vi "sprite.vi"() -> ()   [LabVIEW 2023]
uses:
  data_type/pixel/pixel.ctl
panel:
  in  "mutiply by":u64 min=1 step=1
  in  "exclude color":u32(colorbox)
  out "screen":picture
  in  "save":bool
  in  "sprite name":string
  in  "pixel art":T1
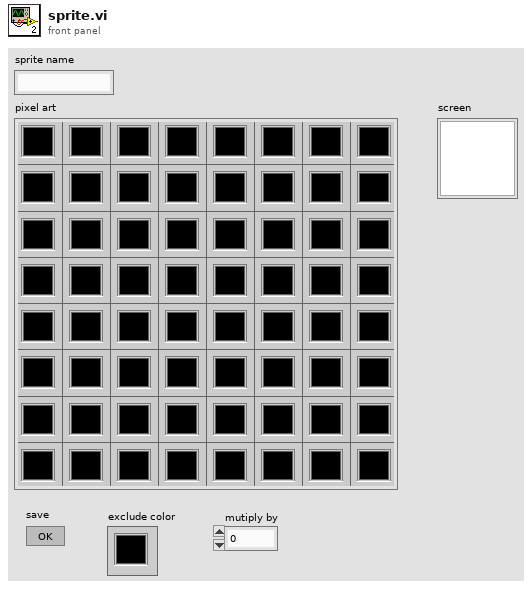
[diagram p1: front panel]
types:
  T1 = cluster{"Color Box":u32, "Color Box 2":u32, "Color Box 3":u32, "Color Box 4":u32, "Color Box 5":u32, "Color Box 6":u32, "Color Box 7":u32, "Color Box 8":u32, "Color Box 9":u32, "Color Box 10":u32, "Color Box 11":u32, "Color Box 12":u32, "Color Box 13":u32, "Color Box 14":u32, "Color Box 15":u32, "Color Box 16":u32, "Color Box 17":u32, "Color Box 18":u32, "Color Box 19":u32, "Color Box 20":u32, "Color Box 21":u32, "Color Box 22":u32, "Color Box 23":u32, "Color Box 24":u32, "Color Box 25":u32, "Color Box 26":u32, "Color Box 27":u32, "Color Box 28":u32, "Color Box 29":u32, "Color Box 30":u32, "Color Box 31":u32, "Color Box 32":u32, "Color Box 33":u32, "Color Box 34":u32, "Color Box 35":u32, "Color Box 36":u32, "Color Box 37":u32, "Color Box 38":u32, "Color Box 39":u32, "Color Box 40":u32, "Color Box 41":u32, "Color Box 42":u32, "Color Box 43":u32, "Color Box 44":u32, "Color Box 45":u32, "Color Box 46":u32, "Color Box 47":u32, "Color Box 48":u32, "Color Box 49":u32, "Color Box 50":u32, "Color Box 51":u32, "Color Box 52":u32, "Color Box 53":u32, "Color Box 54":u32, "Color Box 55":u32, "Color Box 56":u32, "Color Box 57":u32, "Color Box 58":u32, "Color Box 59":u32, "Color Box 60":u32, "Color Box 61":u32, "Color Box 62":u32, "Color Box 63":u32, "Color Box 64":u32}
  T2 = typedef "pixel.ctl" = cluster{"point":cluster{"x":i16, "y":i16}, "Color Box":u32}
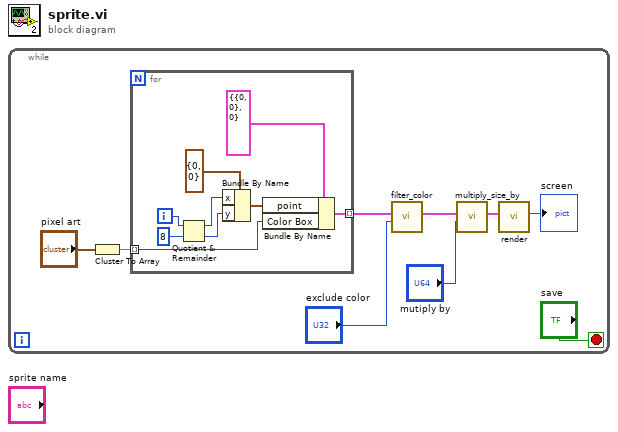
[diagram p0: block diagram]
diagram:
  n1 = while {
    stop <- "save" stop-if-true
    n2 = Cluster To Array(cluster="pixel art") -> (array=w7:u32[])
    n3 = for {
      tunnel: w7 -> [w17] mode=indexing
      tunnel: [w10] -> w4 mode=indexing
      i -> [w14]
      n4 = Quotient & Remainder(x=w14, y=8) -> (x-y*floor(x/y)=w12:i32, floor(x/y)=w11:i32)
      n5 = Bundle By Name(cluster=cluster{"x":i16, "y":i16} {"x"=0, "y"=0} ("point"), "x"=w12, "y"=w11) -> (w15:cluster{"x":i16, "y":i16})
      n6 = Bundle By Name(cluster=T2 {"point"={"x"=0, "y"=0}, "Color Box"=0} ("Pixel"), "point"=w15, "Color Box"=w17) -> (w10:T2)
    }
    n7 = call "filter_color.vi"("exclude color"="exclude color", "input"=w4) -> ("output"=w3:T2[])  [unwired: 9 in]
    n8 = call "multiply_size_by.vi"("mutiply"="mutiply by", "in"=w3) -> ("out"=w2:T2[])  [unwired: 9 in]
    n9 = call "render.vi"("Pixels"=w2) -> ("screen"=→"screen":picture)  [unwired: 10 in]
  }
